vi "CVT String IndexRead.vi"(3 "error in (no error)":errorcluster, 5 "Tag Index":i32) -> (0 "error out":errorcluster, 1 "Value":string)   [LabVIEW 2016]
uses:
  <vilib>/NI/Current Value Table/DataTypes/String_Read Index.vi
  <vilib>/NI/Current Value Table/Memory Block.vi
  <vilib>/NI/Current Value Table/DataTypes/String_Memory Block.vi
  <vilib>/NI/Current Value Table/Current Value Table.lvlib
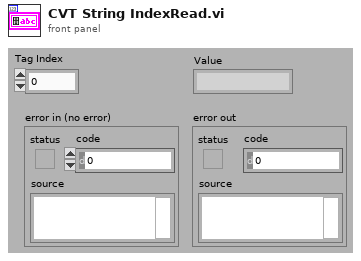
[diagram p1: front panel]
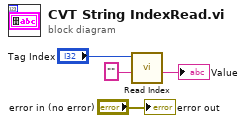
[diagram p0: block diagram]
diagram:
  n1 = call-poly <vilib>:"Read Index.vi"("Default"="", "Index"="Tag Index") -> ("Value"=→"Value":string)  [unwired: 9 in]
  "error out" <- "error in (no error)"
